vi "get_number_points_lidar.vi"(4 "Number lasers":i32=32, 5 "Horizontal_resolution":dbl) -> (2 "Number points":i32)   [LabVIEW 2019]
doc: "Gets the number of points on a data packet depending on the horizontal resolution."
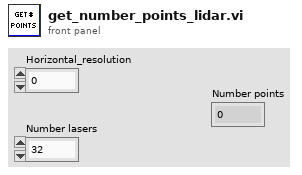
[diagram p1: front panel]
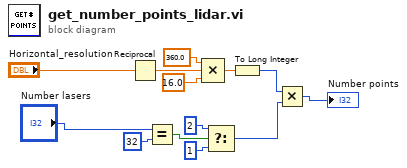
[diagram p0: block diagram]
diagram:
  n1 = Reciprocal(x="Horizontal_resolution") -> (1/x=w12:dbl)
  n2 = Equal?(x="Number lasers", y=32) -> (x = y?=w5:bool)
  n3 = Compound Arithmetic op=MULTIPLY(360.0 ("x"), w12, 16.0 ("value")) -> (w10:dbl)
  n4 = Select(t=2, s=w5, f=1 ("t")) -> (s? t:f=w1:i32)
  n5 = To Long Integer(number=w10) -> (32bit integer=w7:i32)
  n6 = Multiply(x=w7, y=w1) -> (x*y=→"Number points":i32)
